vi "Read Joystick.vi"(8 "Joystick Deadbanded Value (default of 0.1)":dbl, 10 "Joystick R 2 DevRef":T1, 11 "Joystick L 1 DevRef":T1) -> (0 "Wheel Lock":bool=TRUE, 1 "Joystick R 2 X Axis":dbl, 2 "Joystick L 1 Y Axis":dbl, 3 "Joystick L 1 X Axis":dbl, 4 "Radial Spin":bool)   [LabVIEW 2012]
uses:
  <vilib>/Rock Robotics/WPI/Joystick/WPI_JoystickDevRef.ctl
  <vilib>/Rock Robotics/WPI/Joystick/WPI_JoystickDeviceEnum.ctl
  Begin/Global Variables.vi
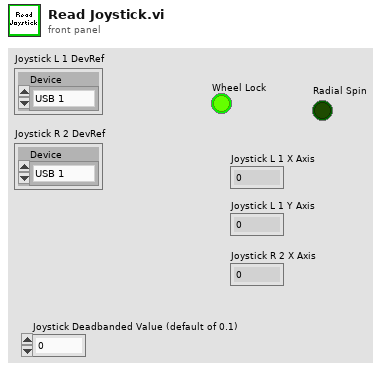
[diagram p1: front panel]
types:
  T1 = typedef "WPI_JoystickDevRef.ctl" = cluster{"Device":T2}
  T2 = typedef "WPI_JoystickDeviceEnum.ctl" = enum16{"USB 1", "USB 2", "USB 3", "USB 4", "Kinect 1", "Kinect 2"}
  T3 = typedef "WPI_JoystickButtonState.ctl" = cluster{"Button 1":bool, "Button 2":bool, "Button 3":bool, "Button 4":bool, "Button 5":bool, "Button 6":bool, "Button 7":bool, "Button 8":bool, "Button 9":bool, "Button 10":bool, "Button 11":bool, "Button 12":bool}
  T4 = cluster{"axis 1 (x)":dbl, "axis 2 (y)":dbl, "axis 3 (throttle)":dbl, "axis 4":dbl, "axis 5":dbl, "axis 6":dbl}
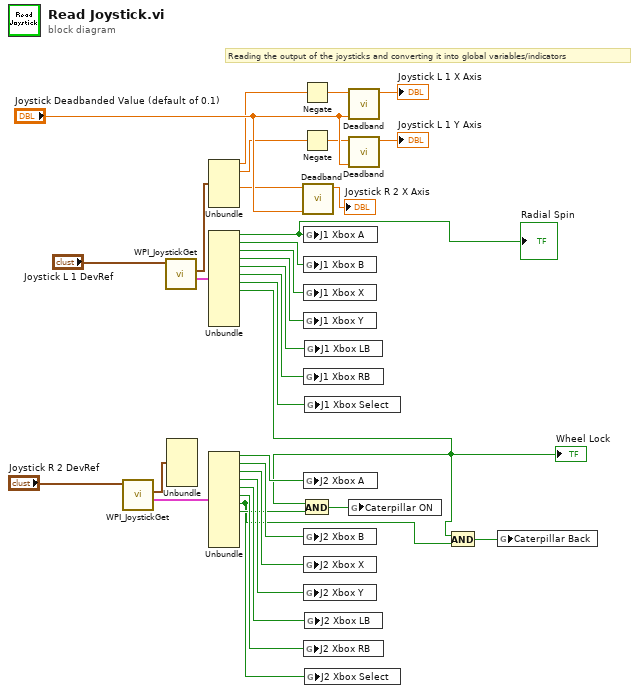
[diagram p0: block diagram]
diagram:
  # "Reading the output of the joysticks and converting it into global variables/indicators"
  n1 = call <vilib>:"WPI_JoystickGet.vi"("JoystickDevRef"="Joystick R 2 DevRef") -> ("Buttons"=w23:T3, "Axes"=w22:T4)  [unwired: 4 in, 1 out]
  n2 = call <vilib>:"WPI_JoystickGet.vi"("JoystickDevRef"="Joystick L 1 DevRef") -> ("Buttons"=w33:T3, "Axes"=w32:T4)  [unwired: 4 in, 1 out]
  n3 = Unbundle(w22) -> ()  [unwired: 6 out]
  n4 = Unbundle(w32) -> ("axis 1 (x)"=w16:dbl, "axis 2 (y)"=w26:dbl, "axis 4"=w8:dbl)  [unwired: 3 out]
  n5 = Unbundle(w33) -> ("Button 1"=w1:bool, "Button 2"=w12:bool, "Button 3"=w18:bool, "Button 4"=w14:bool, "Button 5"=w24:bool, "Button 6"=w25:bool, "Button 7"=w6:bool, "Button 8"=w3:bool)  [unwired: 4 out]
  "Wheel Lock" <- w3
  "Radial Spin" <- w1
  n6 = Unbundle(w23) -> ("Button 1"=w20:bool, "Button 2"=w10:bool, "Button 3"=w13:bool, "Button 4"=w11:bool, "Button 5"=w19:bool, "Button 6"=w9:bool, "Button 7"=w2:bool, "Button 8"=w5:bool)  [unwired: 4 out]
  n7 = Negate(x=w16) -> (-x=w17:dbl)
  n8 = Negate(x=w26) -> (-x=w15:dbl)
  n9 = And(x=w3, y=w5) -> (x .and. y?=w7:bool)
  n10 = call "Deadband.vi"("Value to Deadband (default of 0.1)"="Joystick Deadbanded Value (default of 0.1)", "Value"=w8) -> ("Deadbanded Value"=→"Joystick R 2 X Axis":dbl)  [unwired: 9 in]
  n11 = global write "Global Variables.vi" "J1 Xbox A"(w1) -> ()
  n12 = global write "Global Variables.vi" "J1 Xbox B"(w12) -> ()
  n13 = global write "Global Variables.vi" "J1 Xbox X"(w18) -> ()
  n14 = global write "Global Variables.vi" "J1 Xbox Y"(w14) -> ()
  n15 = global write "Global Variables.vi" "J1 Xbox RB"(w25) -> ()
  n16 = global write "Global Variables.vi" "J2 Xbox A"(w20) -> ()
  n17 = global write "Global Variables.vi" "J2 Xbox B"(w10) -> ()
  n18 = global write "Global Variables.vi" "J2 Xbox X"(w13) -> ()
  n19 = global write "Global Variables.vi" "J2 Xbox Y"(w11) -> ()
  n20 = global write "Global Variables.vi" "J2 Xbox RB"(w9) -> ()
  n21 = global write "Global Variables.vi" "J1 Xbox LB"(w24) -> ()
  n22 = global write "Global Variables.vi" "J1 Xbox Select"(w6) -> ()
  n23 = global write "Global Variables.vi" "J2 Xbox LB"(w19) -> ()
  n24 = global write "Global Variables.vi" "J2 Xbox Select"(w2) -> ()
  n25 = call "Deadband.vi"("Value to Deadband (default of 0.1)"="Joystick Deadbanded Value (default of 0.1)", "Value"=w17) -> ("Deadbanded Value"=→"Joystick L 1 X Axis":dbl)  [unwired: 9 in]
  n26 = call "Deadband.vi"("Value to Deadband (default of 0.1)"="Joystick Deadbanded Value (default of 0.1)", "Value"=w15) -> ("Deadbanded Value"=→"Joystick L 1 Y Axis":dbl)  [unwired: 9 in]
  n27 = global write "Global Variables.vi" "Caterpillar ON"(w7) -> ()
  n28 = And(x=w3, y=w2) -> (x .and. y?=w4:bool)
  n29 = global write "Global Variables.vi" "Caterpillar Back"(w4) -> ()
